vi "GetApplicationSettings.vi"(0 "Application in":refnum<class "Application.lvclass">, 5 "error in (no error)":errorcluster) -> (14 "Application out":refnum<class "Application.lvclass">, 19 "error out":errorcluster)   [LabVIEW 2016, in "Application.lvclass"]
uses:
  Application.lvclass
  Application.lvclass/Application.ctl
  RobotType.ctl
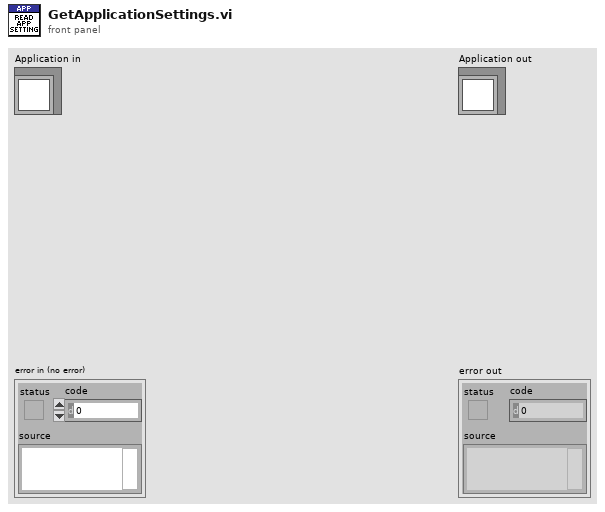
[diagram p1: front panel]
types:
  T1 = typedef "Application.lvclass/RobotType.ctl" = enum16{"UR E-Series", "UR CB-Series"}
  T2 = typedef "NI_LVConfig.lvlib/Config Data RefNum.ctl" = refnum<k1>
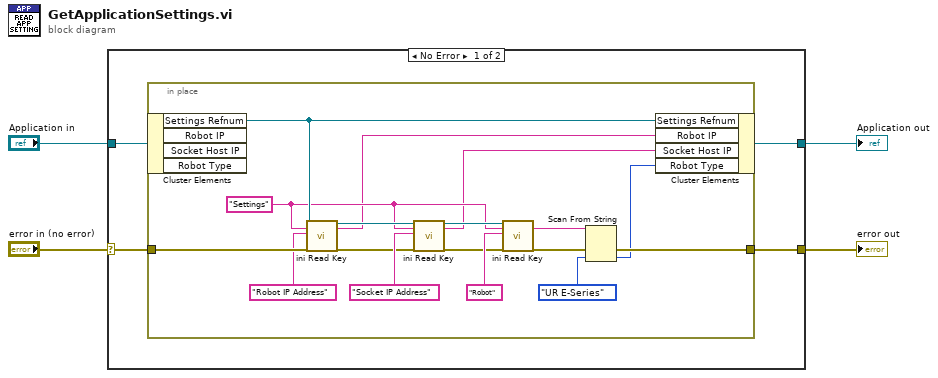
[diagram p0: block diagram]
diagram:
  n1 = case shown="No Error" "error in (no error)" {
    selector: "error in (no error)" -> [w6 w27]
    tunnel: [w5 w27] -> w3
    tunnel: [w7 w26] -> w1
    tunnel: "Application in" -> [w8 w26]
    frame No Error {
      n2 = in-place {
        in-place-border: w6 -> [w25]
        in-place-border: [w20] -> w5
        w13 = "Settings" ("Section")
        n3 = in-place-cluster #1(w8) -> ("Settings Refnum"=w24:T2)  [unwired: 3 out]
        n4 = call "ini Read Key.vi"("Refnum in"=w24, "Section"=w13, "Key"="Robot IP Address", "Error In"=w25) -> ("Refnum out"=w16:T2, "value"=w9:string, "error out"=w10:errorcluster)  [unwired: 13 in]
        n5 = call "ini Read Key.vi"("Refnum in"=w16, "Section"=w13, "Key"="Socket IP Address", "Error In"=w10) -> ("Refnum out"=w15:T2, "value"=w11:string, "error out"=w14:errorcluster)  [unwired: 13 in]
        n6 = call "ini Read Key.vi"("Refnum in"=w15, "Section"=w13, "Key"="Robot", "Error In"=w14) -> ("value"=w17:string, "error out"=w21:errorcluster)  [unwired: 13 in, 1 out]
        n7 = Scan From String(input string=w17, error in=w21, default 1=RobotType."UR E-Series" ("RobotType")) -> (error out=w20:errorcluster, output 1=w18:T1)  [unwired: 2 in, 2 out]
        n8 = in-place-cluster #1("Settings Refnum"=w24, "Robot IP"=w9, "Socket Host IP"=w11, "Robot Type"=w18) -> (w7:refnum<class "Application.lvclass">)
      }
    }
    frame Error {
    }
  }
  "error out" <- w3
  "Application out" <- w1
